vi "FormatUID.vi"(1 "UID":i32) -> (0 "Name":string)   [LabVIEW 2014, in "VI Interpreter.lvclass"]
uses:
  VI Interpreter.lvclass
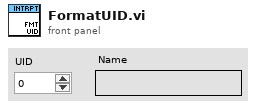
[diagram p1: front panel]
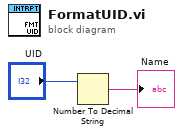
[diagram p0: block diagram]
diagram:
  n1 = Number To Decimal String(number="UID") -> (decimal integer string=→"Name":string)  [unwired: 1 in]
